vi "Read Pin Map v2.vi"(8 "error in (no error)":errorcluster, 11 "NI-DAQ in":refnum<class "NI-DAQ.lvclass">) -> (0 "error out":errorcluster, 2 "Pin Map":T1={"Region Valves"=[49, 52, 0, 0], "Extra Valves"=[[[0.0, 48.0, 0.0, 0.0, 0.0]]], "Tool Primary Valve"=51, "Tool Secondary Valve"=50, "Region Sensors"=[37, 41, 37], "Extra Sensors"=[[[36.0, 37.0, 0.0, 0.0]]], "Tool Primary Sensor"=39.0, "Tool Secondary Sensor"=38.0, "Compression Sensor"=31.0, "5V"=50, "Dispenser Sensor"=0.0}, 3 "NI-DAQ out":refnum<class "NI-DAQ.lvclass">)   [LabVIEW 2021, in "NI-DAQ.lvclass"]
uses:
  NI-DAQ.lvclass
  <vilib>/Utility/file.llb/Read Delimited Spreadsheet (DBL).vi
  I-O.lvclass
  Pin Map.ctl
panel:
  out "extra valves":i32[][][](array[numeric])
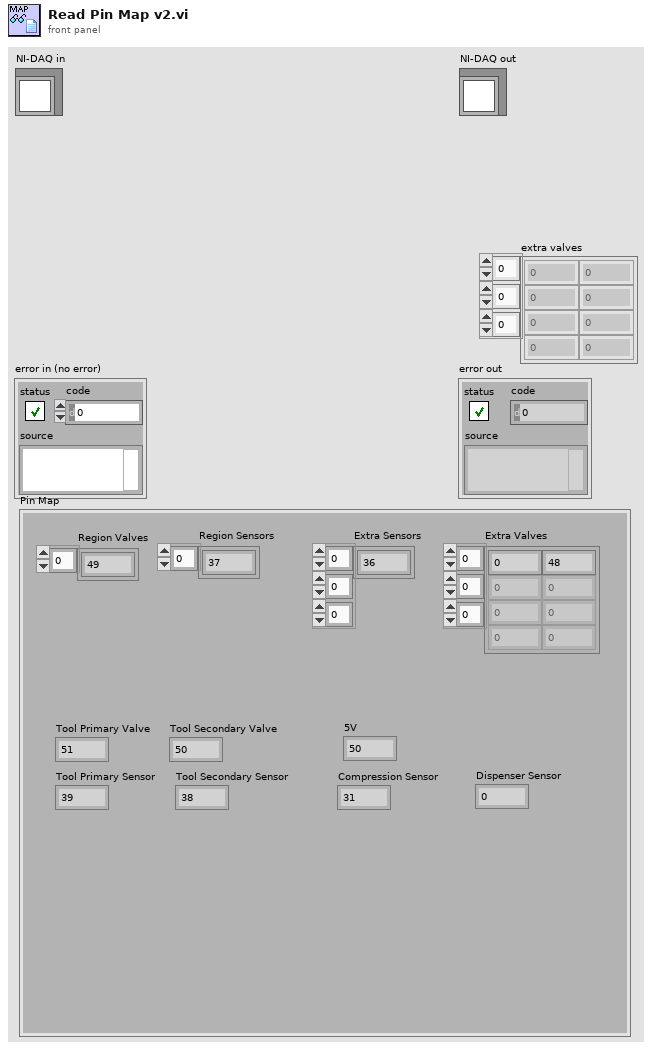
[diagram p1: front panel]
types:
  T1 = typedef "I-O.lvclass/Pin Map.ctl" = cluster{"Region Valves":i32[], "Extra Valves":dbl[][][], "Tool Primary Valve":i32, "Tool Secondary Valve":i32, "Region Sensors":i32[], "Extra Sensors":dbl[][][], "Tool Primary Sensor":dbl, "Tool Secondary Sensor":dbl, "Compression Sensor":dbl, "5V":i32, "Dispenser Sensor":dbl}
  T2 = typedef "File Paths.ctl" = cluster{"Glue Pattern Folder":path, "Carrier Tray Folder":path, "Pick Up Tool Fixture Folder":path, "Components Folder":path, "Bellows Tool Offset.txt":path, "Pick Up Tool Offset.txt":path, "Dispense Tip Offset.txt":path, "Log Files":path, "Gantry Assembly Map.txt":path, "Syringe and offset map.txt":path, "Controllers Folder":path, "Local dbase config":path}
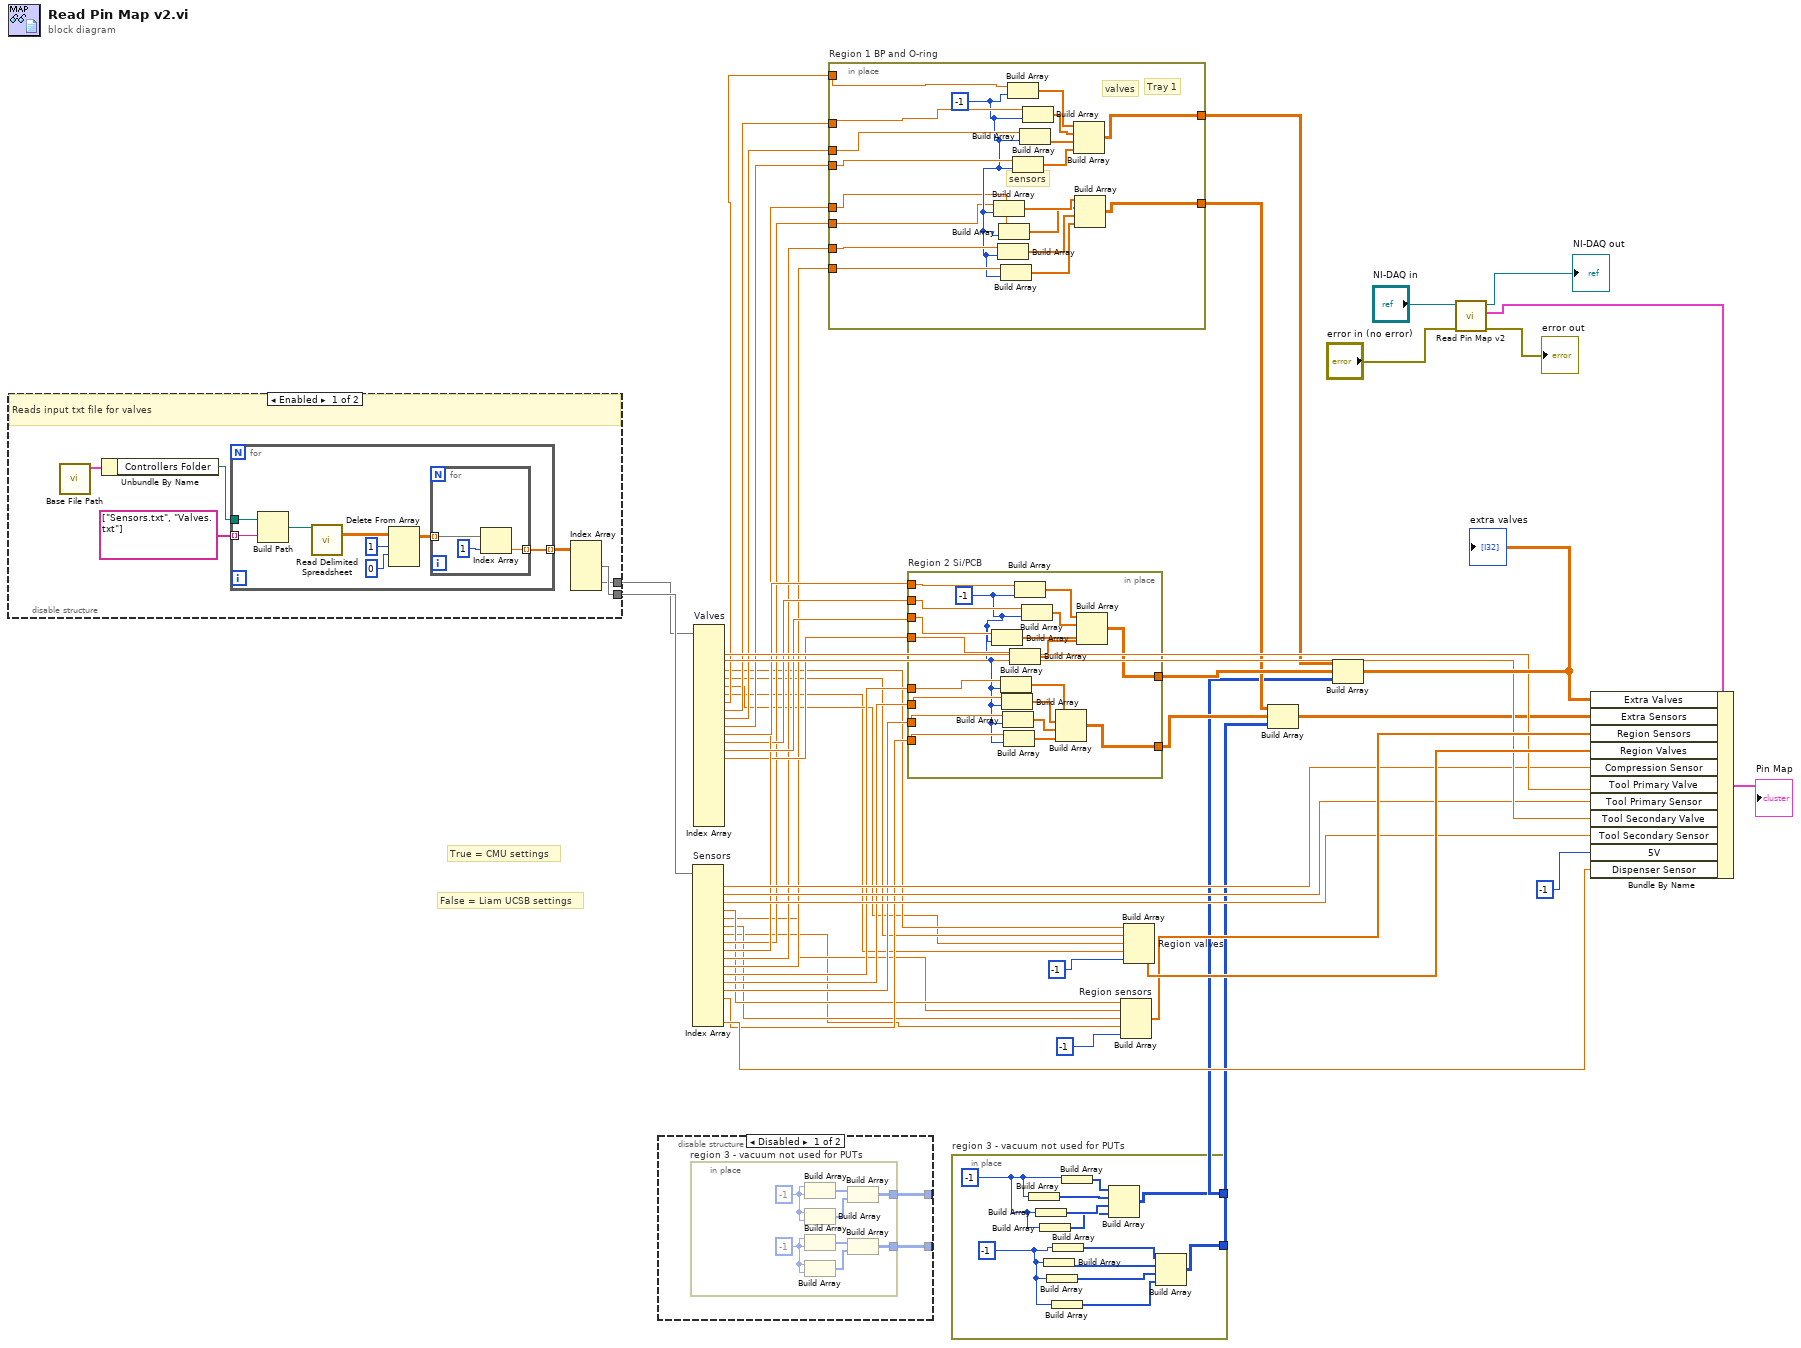
[diagram p0: block diagram]
diagram:
  # "False = Liam UCSB settings"
  # "True = CMU settings"
  n1 = disable-structure shown="Enabled" {
    disable-tunnel: [w53 _] -> w51
    disable-tunnel: [w52 _] -> w50
    frame Enabled {
      # "Reads input txt file for valves"
      n2 = call "Base File Path.vi"() -> ("Paths Out"=w57:T2)  [unwired: 11 in]
      n3 = Unbundle By Name(w57) -> ("Controllers Folder"=w55:path)
      n4 = for {
        tunnel: string[] ["Sensors.txt", "Valves.txt"] -> [w63] mode=indexing
        tunnel: w55 -> [w64]
        tunnel: [w58] -> w54 mode=indexing
        n5 = Build Path(base path=w64, name or relative path=w63) -> (appended path=w65:path)
        n6 = call-poly <vilib>:"Read Delimited Spreadsheet.vi"("file path (dialog if empty)"=w65) -> ("all rows"=w62:dbl[][])  [unwired: 9 in, 5 out]
        n7 = Delete From Array(array=w62, length=1, index (row)=0) -> (array with subset deleted=w59:dbl[][])  [unwired: 1 in, 1 out]
        n8 = for {
          tunnel: w59 -> [w68] mode=indexing
          tunnel: [w67] -> w58 mode=indexing
          n9 = Index Array(array=w68, index=1) -> (element=w67:dbl)
        }
      }
      n10 = Index Array(array=w54) -> (element #1=w53:dbl[], element #2=w52:dbl[])  [unwired: 4 in]
    }
    frame Disabled {
    }
  }
  n11 = disable-structure shown="Disabled" {
    disable-tunnel: [w70 _] -> _
    disable-tunnel: [w69 _] -> _
    frame Disabled {
      n12 = in-place "region 3 - vacuum not used for PUTs" {
        in-place-border: [w75] -> w70
        in-place-border: [w72] -> w69
        w71 = -1
        w77 = -1
        n13 = Build Array "Build Array"(w77, w77) -> (w78:i32[])
        n14 = Build Array(w77, w77) -> (w76:i32[])
        n15 = Build Array(w71, w71) -> (w74:i32[])
        n16 = Build Array(w71, w71) -> (w73:i32[])
        n17 = Build Array(w78, w76) -> (w75:i32[][])
        n18 = Build Array(w74, w73) -> (w72:i32[][])
      }
    }
    frame Enabled {
    }
  }
  n19 = Index Array "Sensors"(array=w51) -> (element #1=w36:dbl, element #2=w35:dbl, element #3=w34:dbl, element #4=w4:dbl, element #5=w3:dbl, element #6=w2:dbl, element #7=w1:dbl, element #8=w15:dbl, element #9=w23:dbl, element #10=w14:dbl, element #11=w13:dbl, element #12=w12:dbl, element #13=w9:dbl, element #14=w10:dbl, element #15=w11:dbl, element #18=w22:dbl)  [unwired: 18 in, 2 out]
  n20 = Index Array "Valves"(array=w50) -> (element #2=w38:dbl, element #3=w37:dbl, element #4=w8:dbl, element #5=w7:dbl, element #6=w6:dbl, element #7=w5:dbl, element #8=w29:dbl, element #9=w28:dbl, element #10=w18:dbl, element #11=w27:dbl, element #12=w26:dbl, element #13=w17:dbl, element #14=w25:dbl, element #15=w16:dbl)  [unwired: 23 in, 9 out]
  n21 = in-place "Region 1 BP and O-ring" {
    in-place-border: [w97] -> w33
    in-place-border: [w96] -> w31
    in-place-border: w29 -> [w95]
    in-place-border: w28 -> [w89]
    in-place-border: w27 -> [w87]
    in-place-border: w23 -> [w79]
    in-place-border: w18 -> [w88]
    in-place-border: w15 -> [w80]
    in-place-border: w14 -> [w85]
    in-place-border: w13 -> [w82]
    w81 = -1
    # "sensors"
    # "valves"
    # "Tray 1"
    n22 = Build Array(w80, w81) -> (w90:dbl[])
    n23 = Build Array(w85, w81) -> (w84:dbl[])
    n24 = Build Array(w79, w81) -> (w86:dbl[])
    n25 = Build Array(w82, w81) -> (w83:dbl[])
    n26 = Build Array(w95, w81) -> (w94:dbl[])
    n27 = Build Array(w87, w81) -> (w91:dbl[])
    n28 = Build Array(w88, w81) -> (w92:dbl[])
    n29 = Build Array(w89, w81) -> (w93:dbl[])
    n30 = Build Array(w94, w93, w92, w91) -> (w97:dbl[][])
    n31 = Build Array(w90, w86, w84, w83) -> (w96:dbl[][])
  }
  n32 = in-place "Region 2 Si/PCB" {
    in-place-border: [w116] -> w32
    in-place-border: [w115] -> w30
    in-place-border: w26 -> [w110]
    in-place-border: w25 -> [w108]
    in-place-border: w17 -> [w109]
    in-place-border: w16 -> [w107]
    in-place-border: w12 -> [w106]
    in-place-border: w11 -> [w104]
    in-place-border: w10 -> [w102]
    in-place-border: w9 -> [w100]
    w98 = -1
    n33 = Build Array(w108, w98) -> (w113:dbl[])
    n34 = Build Array(w106, w98) -> (w105:dbl[])
    n35 = Build Array(w100, w98) -> (w99:dbl[])
    n36 = Build Array(w102, w98) -> (w101:dbl[])
    n37 = Build Array(w104, w98) -> (w103:dbl[])
    n38 = Build Array(w107, w98) -> (w114:dbl[])
    n39 = Build Array(w110, w98) -> (w111:dbl[])
    n40 = Build Array(w109, w98) -> (w112:dbl[])
    n41 = Build Array(w105, w99, w101, w103) -> (w115:dbl[][])
    n42 = Build Array(w111, w112, w113, w114) -> (w116:dbl[][])
  }
  n43 = in-place "region 3 - vacuum not used for PUTs" {
    in-place-border: [w128] -> w21
    in-place-border: [w127] -> w20
    w118 = -1
    w123 = -1
    n44 = Build Array(w123) -> (w125:i32[])
    n45 = Build Array(w123) -> (w124:i32[])
    n46 = Build Array(w123) -> (w122:i32[])
    n47 = Build Array(w118) -> (w119:i32[])
    n48 = Build Array(w118) -> (w120:i32[])
    n49 = Build Array(w118) -> (w117:i32[])
    n50 = Build Array(w118) -> (w121:i32[])
    n51 = Build Array(w123) -> (w126:i32[])
    n52 = Build Array(w126, w125, w124, w122) -> (w128:i32[][])
    n53 = Build Array(w121, w119, w120, w117) -> (w127:i32[][])
  }
  n54 = Build Array "Region sensors"(w4, w3, w2, w1, -1) -> (w41:dbl[])
  n55 = Build Array "Region valves"(w8, w7, w6, w5, -1) -> (w43:dbl[])
  n56 = Build Array(w31, w30, w20) -> (w19:dbl[][][])
  n57 = Build Array(w33, w32, w21) -> (w40:dbl[][][])
  "extra valves" <- w40
  n58 = call-parent "Read Pin Map v2.vi"("error in (no error)"="error in (no error)", "I-O in"="NI-DAQ in") -> ("error out"=→"error out":errorcluster, "Pin Map 2"=w45:T1, "I-O out"=→"NI-DAQ out":refnum<class "NI-DAQ.lvclass">)  [unwired: 7 in]
  n59 = Bundle By Name(cluster=w45, "Extra Valves"=w40, "Extra Sensors"=w19, "Region Sensors"=w41, "Region Valves"=w43, "Compression Sensor"=w36, "Tool Primary Valve"=w38, "Tool Primary Sensor"=w35, "Tool Secondary Valve"=w37, "Tool Secondary Sensor"=w34, "5V"=-1, "Dispenser Sensor"=w22) -> (→"Pin Map":T1)
